vi "Write Log Level.vi"(10 "log level":T1=enum."None", 11 "connection in":refnum<class "Low Level Connection.lvclass">) -> (3 "connection out":refnum<class "Low Level Connection.lvclass">)   [LabVIEW 2020, in "NI_SFTP.lvlib" / "Low Level Connection.lvclass"]
uses:
  <vilib>/net/SFTP/Low Level Connection/Low Level Connection.lvclass
  <vilib>/net/SFTP/Low Level Connection/Log Level.ctl
  <vilib>/net/SFTP/Low Level Connection/Low Level Connection.lvclass/Low Level Connection.ctl
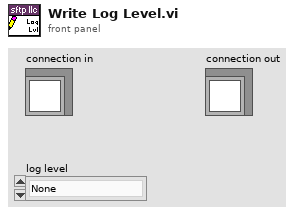
[diagram p1: front panel]
types:
  T1 = typedef "NI_SFTP.lvlib/Low Level Connection.lvclass/Log Level.ctl" = enum16{"Debug", "Information", "Warning", "Error", "None"}
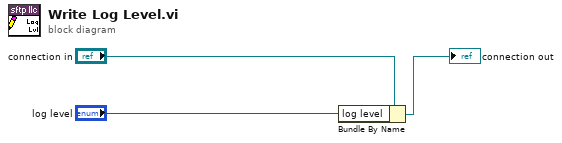
[diagram p0: block diagram]
diagram:
  n1 = Bundle By Name(cluster="connection in", "log level"="log level") -> (→"connection out":refnum<class "Low Level Connection.lvclass">)
